vi "Get Result.vi"(11 "Log Preparer Module in":refnum<class "Log Preparer Module.lvclass">) -> (2 "error out":errorcluster, 3 "Result":T1, 5 "Log":string)   [LabVIEW 2020, in "VolatusData.lvlib" / "Log Preparer Module.lvclass"]
uses:
  Log Preparer Module.lvclass
  Log Preparer Module.lvclass/Log Preparer Module.ctl
  Prep State.ctl
  VolatusData.lvlib
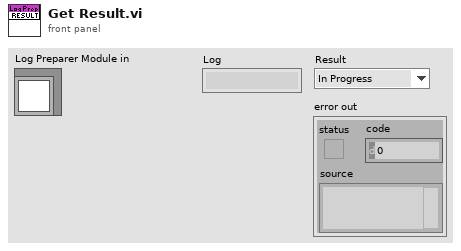
[diagram p1: front panel]
types:
  T1 = typedef "VolatusData.lvlib/Prep State.ctl" = enum16{"In Progress", "Success", "Failed"}
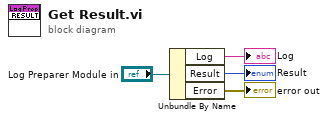
[diagram p0: block diagram]
diagram:
  n1 = Unbundle By Name("Log Preparer Module in") -> ("Log"=→"Log":string, "Result"=→"Result":T1, "Error"=→"error out":errorcluster)
